vi "FM_Tx_Template.vi"() -> ()   [LabVIEW 2013]
uses:
  <vilib>/measure/NI_MAPro.lvlib
  <instrlib>/niUSRP/niUSRP Write Tx Data (CDB Cluster).vi
  <vilib>/Analysis/NI_AALBase.lvlib
  <vilib>/Analysis/baseanly.llb/Quick Scale 1D.vi
  <vilib>/measure/maspectr.llb/FFT Power Spectrum and PSD for 1 Chan.vi
  <vilib>/Analysis/3filter.llb/IIR Filter (DBL).vi
panel:
  out "Frequency Modulated Signal Spectrum":dbl[](graph)
  out "Frequency Modulated Signal":dbl[](graph)
  out "Message Specturm":dbl[](graph)
  out "Message":waveform(dbl)(graph)
  out "Error out":errorcluster
  in  "stop":bool
  in  "Peak Deviation (Hz)":dbl=inf min=inf
  in  "# Tones":i32=3
  in  "Delta Frequency":dbl=1000.0 format="%.2p"
  in  "Start Frequency":dbl=1000.0 format="%.2p"
  in  "Message Length\n(samples)":dbl=200000.0
  in  "Active Antenna":string(combo)="TX1"
  out "Actual Gain (dB)":dbl format="%#_6f"
  in  "Gain (dB)":dbl=20.0 min=0.0 max=31.0 format="%#_6f"
  out "Actual Frequency":dbl=100000.0 format="%#_6p"
  in  "Carrier Frequency":dbl=915100000.0 format="%#_6p"
  out "Actual IQ Rate":dbl=100000.0 format="%#_6p"
  in  "IQ Rate":dbl=200000.0 format="%#_6p"
  in  "Device Names":refnum<k15>="192.168.10.2"
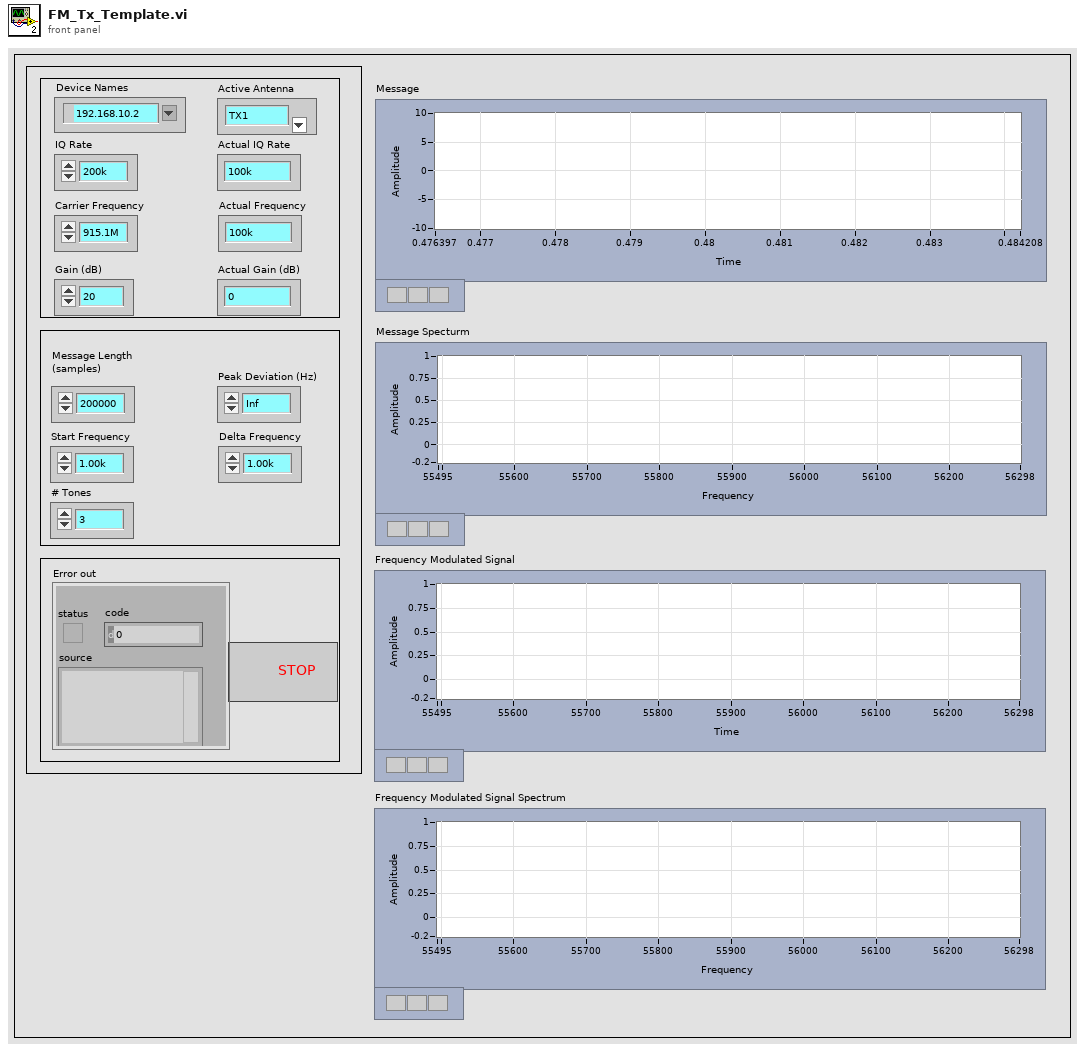
[diagram p1: front panel]
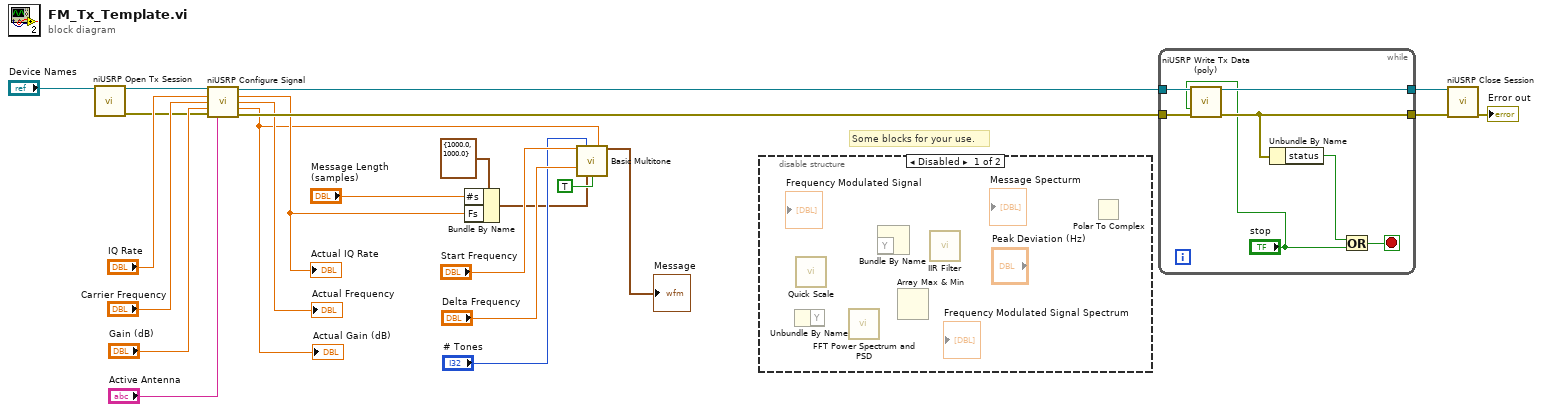
[diagram p0: block diagram]
diagram:
  # "Some blocks for your use."
  n1 = call <instrlib>:"niUSRP Open Tx Session.vi"("device names"="Device Names") -> ("session handle out"=w22:refnum<k15>, "error out"=w18:errorcluster)  [unwired: 13 in]
  n2 = call <instrlib>:"niUSRP Configure Signal.vi"("session handle"=w22, "IQ rate"="IQ Rate", "carrier frequency"="Carrier Frequency", "gain"="Gain (dB)", "error in (no error)"=w18, "active antenna"="Active Antenna") -> ("session handle out"=w12:refnum<k15>, "coerced IQ rate"=w4:dbl, "coerced carrier frequency"=→"Actual Frequency":dbl, "coerced gain"=w1:dbl, "error out"=w10:errorcluster)  [unwired: 5 in]
  "Actual IQ Rate" <- w4
  "Actual Gain (dB)" <- w1
  n3 = Bundle By Name(cluster=cluster{"Fs":dbl, "#s":dbl} {"Fs"=1000.0, "#s"=1000.0} ("sampling info"), "#s"="Message Length\n(samples)", "Fs"=w4) -> (w5:cluster{"Fs":dbl, "#s":dbl})
  n4 = call <vilib>:"Basic Multitone.vi"("start frequency"="Start Frequency", "#tones"="# Tones", "amplitude"=w1, "delta frequency"="Delta Frequency", "sampling info"=w5, "coerce frequencies?"=TRUE) -> ("signal out"=→"Message":waveform(dbl))  [unwired: 6 in, 3 out]
  n5 = disable-structure shown="Disabled" {
    frame Disabled {
      n6 = Unbundle By Name() -> ()  [unwired: 1 in, 1 out]
      n7 = call-poly <vilib>:"Quick Scale.vi"() -> ()  [unwired: 1 in, 3 out]
      n8 = call-poly <vilib>:"FFT Power Spectrum and PSD.vi"() -> ()  [unwired: 8 in, 4 out]
      n9 = Bundle By Name() -> ()  [unwired: 2 in, 1 out]
      n10 = Array Max & Min() -> ()  [unwired: 1 in, 4 out]
      n11 = call-poly <vilib>:"IIR Filter.vi"() -> ()  [unwired: 4 in, 2 out]
      n12 = Polar To Complex() -> ()  [unwired: 2 in, 1 out]
    }
    frame Enabled {
    }
  }
  n13 = while {
    tunnel: w12 -> [w30]
    tunnel: [w29] -> w11
    tunnel: w10 -> [w28]
    tunnel: [w27] -> w7
    stop <- w25 stop-if-true
    n14 = call-poly <instrlib>:"niUSRP Write Tx Data (poly).vi"("session handle"=w30, "end of data?"="stop", "error in (no error)"=w28) -> ("session handle out"=w29:refnum<k15>, "error out"=w27:errorcluster)  [unwired: 11 in]
    n15 = Unbundle By Name(w27) -> ("status"=w26:bool)
    n16 = Or(x=w26, y="stop") -> (x .or. y?=w25:bool)
  }
  n17 = call <instrlib>:"niUSRP Close Session.vi"("session handle"=w11, "error in (no error)"=w7) -> ("error out"=→"Error out":errorcluster)  [unwired: 13 in]
